vi "menuBarSelection.vi"(8 "error in (no error)":errorcluster, 10 "itemPath":string, 11 "ScriptEditorV2 in":refnum<class "ScriptEditorV2.lvclass">) -> (0 "error out":errorcluster, 2 "close":bool, 3 "ScriptEditorV2 out":refnum<class "ScriptEditorV2.lvclass">)   [LabVIEW 2011, in "Views.lvlib" / "ScriptEditor.lvlib" / "ScriptEditorV2.lvclass"]
uses:
  ScriptEditorV2.lvclass
  ScriptEditorV2.lvclass/ScriptEditorV2.ctl
  Tools/DatabaseHelpers.lvlib
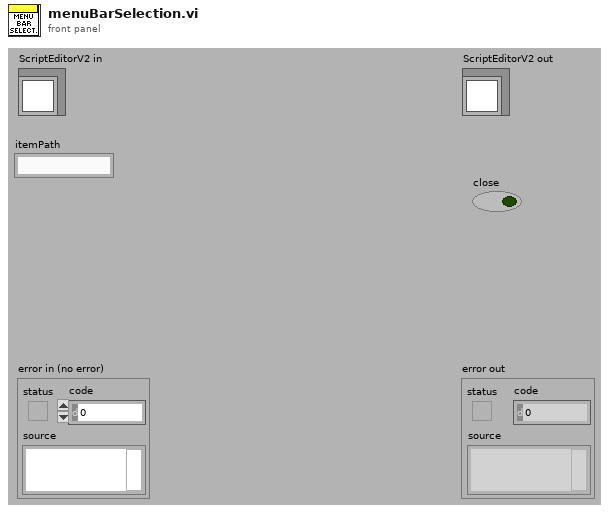
[diagram p1: front panel]
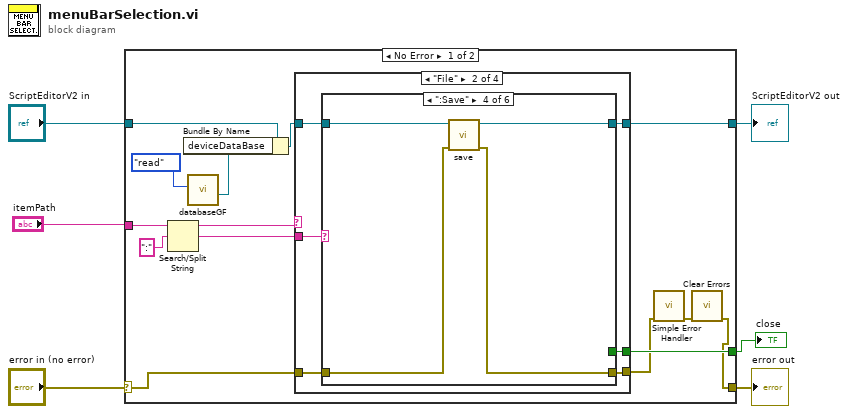
[diagram p0: block diagram]
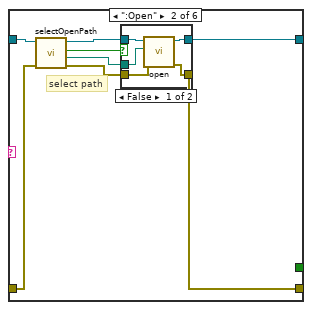
[diagram p4: hidden frame]
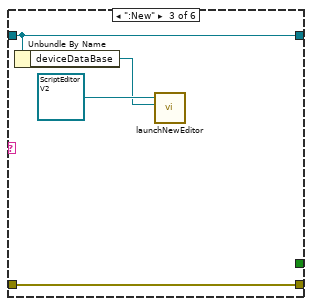
[diagram p6: hidden frame]
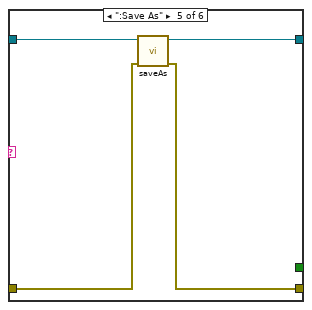
[diagram p7: hidden frame]
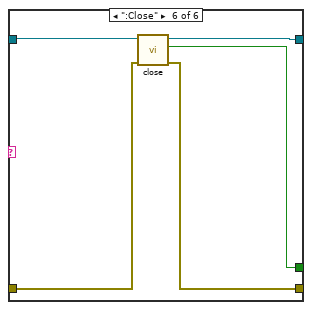
[diagram p8: hidden frame]
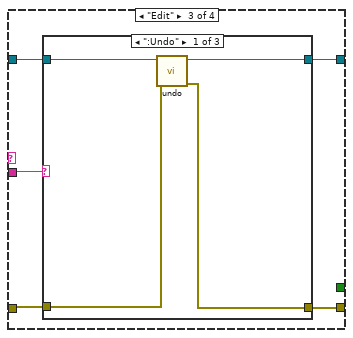
[diagram p9: hidden frame]
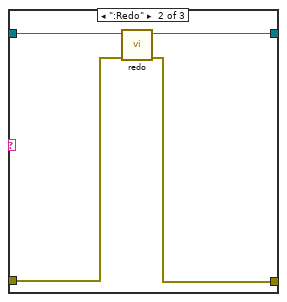
[diagram p10: hidden frame]
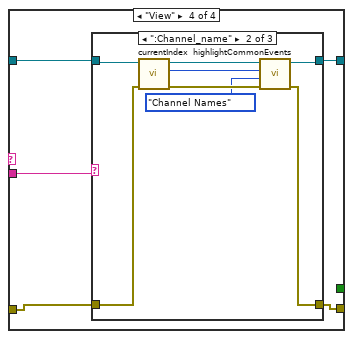
[diagram p12: hidden frame]
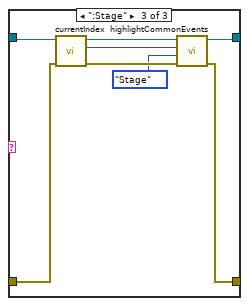
[diagram p14: hidden frame]
diagram:
  n1 = case shown="No Error" "error in (no error)" {
    selector: "error in (no error)" -> [w18 w102]
    tunnel: [w7 w102] -> w5
    tunnel: [w15 w101] -> w3
    tunnel: "ScriptEditorV2 in" -> [w11 w101]
    tunnel: "itemPath" -> [w19 _]
    tunnel: [w14 _] -> w1
    frame No Error {
      n2 = Search/Split String(string=w19, search string/char (-)=":") -> (substring before match=w17:string, match + rest of string=w16:string)  [unwired: 1 in, 1 out]
      n3 = call "databaseGF.vi"("Enum"=enum16{"write", "read"}."read") -> ("deviceDataBase out"=w12:refnum<class "deviceDataBase.lvclass">)  [unwired: 10 in]
      n4 = Bundle By Name(cluster=w11, "deviceDataBase"=w12) -> (w10:refnum<class "ScriptEditorV2.lvclass">)
      n5 = case shown="\"File\"" w17 {
        tunnel: w18 -> [w21 w28 w64 w79]
        tunnel: [w21 w27 w63 w78] -> w8
        tunnel: w16 -> [_ w24 w67 w80]
        tunnel: w10 -> [w22 w26 w66 w82]
        tunnel: [w22 w25 w65 w81] -> w15
        tunnel: [_ w23 _ _] -> w14
        frame Default {
        }
        frame "File" {
          n6 = case shown="\":Save\"" w24 {
            tunnel: w28 -> [w29 w31 w49 w51 w55 w60]
            tunnel: [w29 w37 w49 w50 w54 w59] -> w27
            tunnel: w26 -> [w30 w36 w47 w53 w57 w62]
            tunnel: [w30 w38 w47 w52 w56 w61] -> w25
            tunnel: [_ _ _ _ _ w58] -> w23
            frame Default {
            }
            frame ":Open" {
              # "select path"
              n7 = call "selectOpenPath.vi"("error in (no error)"=w31, "ScriptEditorV2 in"=w36) -> ("error out"=w32:errorcluster, "selected path"=w34:path, "notSelected?"=w33:bool, "ScriptEditorV2 out"=w35:refnum<class "ScriptEditorV2.lvclass">)  [unwired: 6 in]
              n8 = case shown="False" w33 {
                tunnel: [w43 w45] -> w38
                tunnel: w32 -> [w42 w44]
                tunnel: [w41 w44] -> w37
                tunnel: w35 -> [w40 w45]
                tunnel: w34 -> [w39 _]
                frame False {
                  n9 = call "open.vi"("error in (no error)"=w42, "Path"=w39, "ScriptEditorV2 in"=w40) -> ("error out"=w41:errorcluster, "ScriptEditorV2 out"=w43:refnum<class "ScriptEditorV2.lvclass">)  [unwired: 7 in]
                }
                frame True {
                }
              }
            }
            frame ":New" {
              n10 = Unbundle By Name(w47) -> ("deviceDataBase"=w46:refnum<class "deviceDataBase.lvclass">)
              n11 = call-dynamic "launchNewEditor.vi"("deviceDataBase"=w46, "ScriptEditorV2 in"=refnum<class "ScriptEditorV2.lvclass"> refnum ("ScriptEditorV2 in 2")) -> ()  [unwired: 8 in, 2 out]
            }
            frame ":Save" {
              n12 = call "save.vi"("error in (no error)"=w51, "ScriptEditorV2 in"=w53) -> ("error out"=w50:errorcluster, "ScriptEditorV2 out"=w52:refnum<class "ScriptEditorV2.lvclass">)  [unwired: 8 in]
            }
            frame ":Save As" {
              n13 = call "saveAs.vi"("error in (no error)"=w55, "ScriptEditorV2 in"=w57) -> ("error out"=w54:errorcluster, "ScriptEditorV2 out"=w56:refnum<class "ScriptEditorV2.lvclass">)  [unwired: 8 in]
            }
            frame ":Close" {
              n14 = call "close.vi"("error in (no error)"=w60, "ScriptEditorV2 in"=w62) -> ("error out"=w59:errorcluster, "close"=w58:bool, "ScriptEditorV2 out"=w61:refnum<class "ScriptEditorV2.lvclass">)  [unwired: 7 in]
            }
          }
        }
        frame "Edit" {
          n15 = case shown="\":Undo\"" w67 {
            tunnel: w66 -> [w71 w75 w77]
            tunnel: [w70 w74 w77] -> w65
            tunnel: w64 -> [w69 w73 w76]
            tunnel: [w68 w72 w76] -> w63
            frame ":Undo" {
              n16 = call "undo.vi"("error in (no error)"=w69, "ScriptEditorV2 in"=w71) -> ("error out"=w68:errorcluster, "ScriptEditorV2 out"=w70:refnum<class "ScriptEditorV2.lvclass">)  [unwired: 8 in]
            }
            frame ":Redo" {
              n17 = call "redo.vi"("error in (no error)"=w73, "ScriptEditorV2 in"=w75) -> ("error out"=w72:errorcluster, "ScriptEditorV2 out"=w74:refnum<class "ScriptEditorV2.lvclass">)  [unwired: 8 in]
            }
            frame Default {
            }
          }
        }
        frame "View" {
          n18 = case shown="\":Channel_name\"" w80 {
            tunnel: w82 -> [w84 w90 w98]
            tunnel: [w84 w92 w100] -> w81
            tunnel: w79 -> [w83 w86 w94]
            tunnel: [w83 w91 w99] -> w78
            frame Default {
            }
            frame ":Channel_name" {
              n19 = call "currentIndex.vi"("error in (no error)"=w86, "ScriptEditorV2 in"=w90) -> ("error out"=w87:errorcluster, "index"=w88:i32, "ScriptEditorV2 out"=w89:refnum<class "ScriptEditorV2.lvclass">)  [unwired: 7 in]
              n20 = call "highlightCommonEvents.vi"("error in (no error)"=w87, "Enum"=enum16{"Channel Names", "Stage"}."Channel Names", "rowIndex"=w88, "ScriptEditorV2 in"=w89) -> ("error out"=w91:errorcluster, "ScriptEditorV2 out"=w92:refnum<class "ScriptEditorV2.lvclass">)  [unwired: 6 in]
            }
            frame ":Stage" {
              n21 = call "currentIndex.vi"("error in (no error)"=w94, "ScriptEditorV2 in"=w98) -> ("error out"=w95:errorcluster, "index"=w96:i32, "ScriptEditorV2 out"=w97:refnum<class "ScriptEditorV2.lvclass">)  [unwired: 7 in]
              n22 = call "highlightCommonEvents.vi"("error in (no error)"=w95, "Enum"=enum16{"Channel Names", "Stage"}."Stage", "rowIndex"=w96, "ScriptEditorV2 in"=w97) -> ("error out"=w99:errorcluster, "ScriptEditorV2 out"=w100:refnum<class "ScriptEditorV2.lvclass">)  [unwired: 6 in]
            }
          }
        }
      }
      n23 = call <vilib>:"Simple Error Handler.vi"("error in (no error)"=w8) -> ("error out"=w9:errorcluster)  [unwired: 4 in, 4 out]
      n24 = call <vilib>:"Clear Errors.vi"("error in (no error)"=w9) -> ("error out"=w7:errorcluster)  [unwired: 6 in]
    }
    frame Error {
    }
  }
  "error out" <- w5
  "ScriptEditorV2 out" <- w3
  "close" <- w1
